vi "Rotations in cycle to scaling values.vi"(11 "rotations in a cycle":u16) -> (1 "degrees of one u16":dbl, 2 "angle to u16 scale factor":dbl, 3 "total angle span (degrees)":u16)   [LabVIEW 2020, in "Engine Simulation Toolkit System Explorer.lvlib"]
uses:
  Engine Simulation Toolkit System Explorer.lvlib
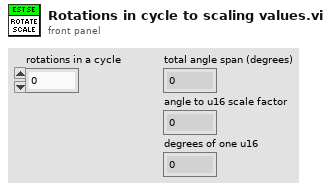
[diagram p1: front panel]
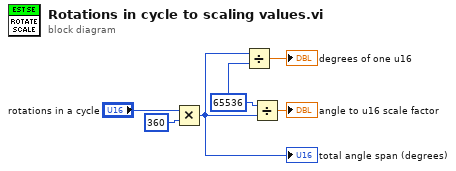
[diagram p0: block diagram]
diagram:
  w2 = u32 65536 ("y")
  n1 = Multiply(x="rotations in a cycle", y=u16 360) -> (x*y=w3:u16)
  "total angle span (degrees)" <- w3
  n2 = Divide(x=w3, y=w2) -> (x/y=→"degrees of one u16":dbl)
  n3 = Divide(x=w2, y=w3) -> (x/y=→"angle to u16 scale factor":dbl)
